vi "Buffer CORE.vi"(5 "Parameters":T3={"Index"=0, "Size"=3000, "Samples"=0, "Ordered ?"=FALSE}, 7 "Mode":T2, 8 "Error IN":errorcluster, 10 "DATA IN":T1[](array[typedef])) -> (0 "Error OUT":errorcluster, 2 "DATA OUT":T1[](array[typedef]), 3 "New Element ?":bool, 4 "Index":i32)   [LabVIEW 2017, in "PMU data buffer.lvlib"]
uses:
  PMU data buffer.lvlib
  Buffer Settings.ctl
  Buffer state.ctl
  Buffer DATA cluster.ctl
panel:
  # "Buffer Paremeters"
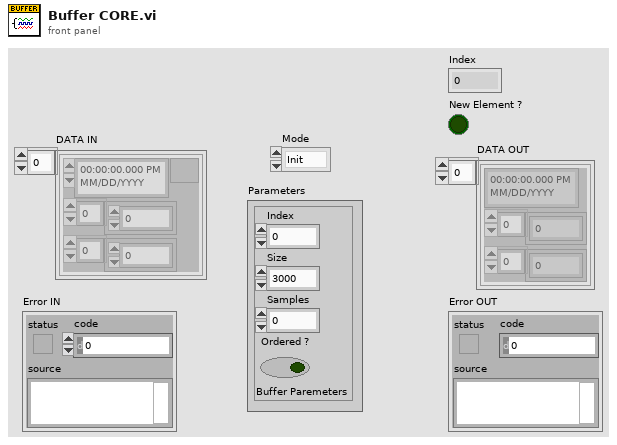
[diagram p1: front panel]
types:
  T1 = typedef "PMU data buffer.lvlib/Buffer DATA cluster.ctl" = cluster{timestamp, csg[], sgl[]}
  T2 = typedef "PMU data buffer.lvlib/Buffer state.ctl" = enum16{"Init", "Change Size", "Flush", "Exit", "Add", "Get", "Hist_Toggle", "Add_Serv"}
  T3 = typedef "PMU data buffer.lvlib/Buffer Settings.ctl" = cluster{"Index":i32, "Size":i32, "Samples":i32, "Ordered ?":bool}
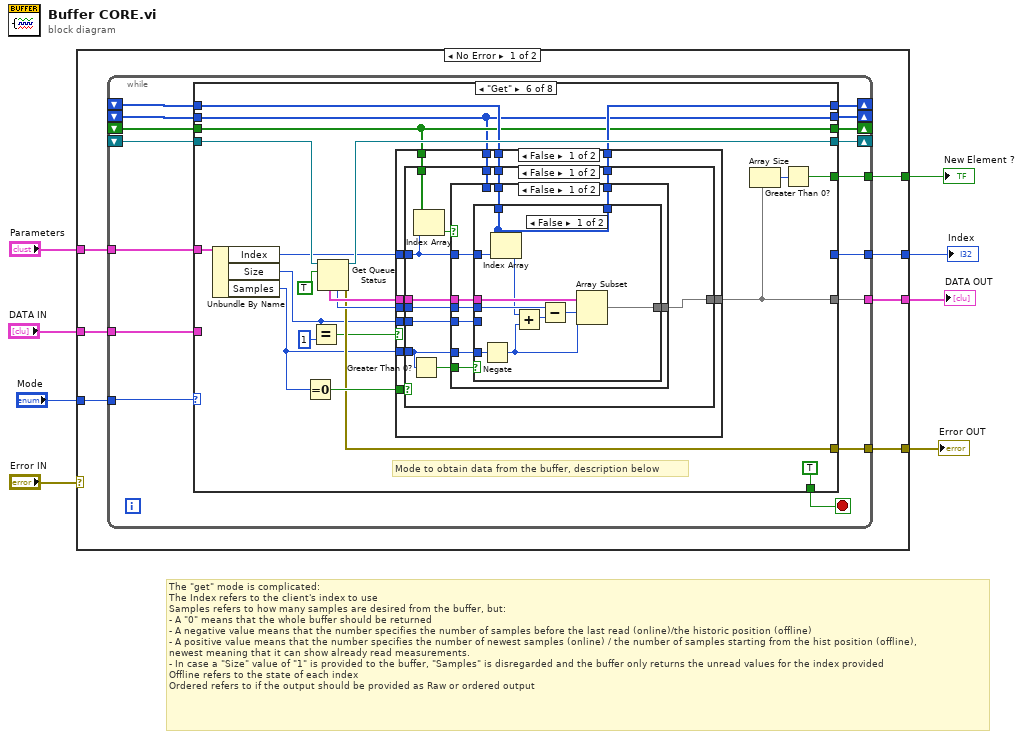
[diagram p0: block diagram]
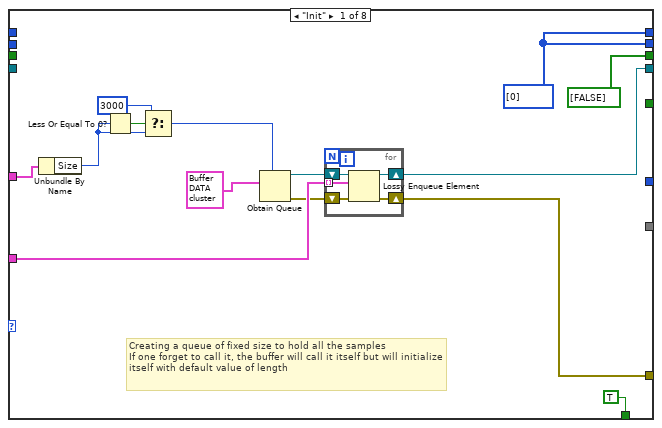
[diagram p2: hidden frame]
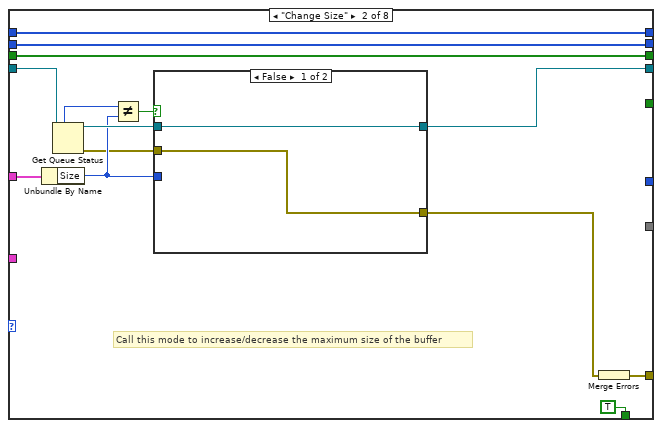
[diagram p3: hidden frame]
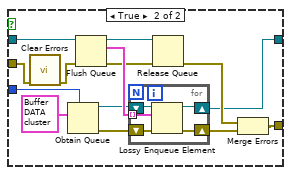
[diagram p4: hidden frame]
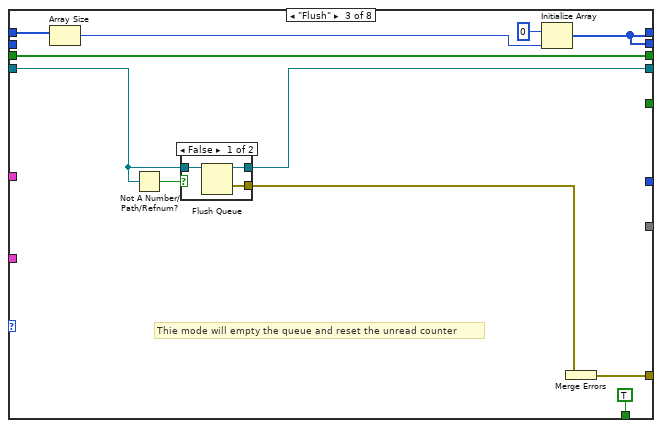
[diagram p5: hidden frame]
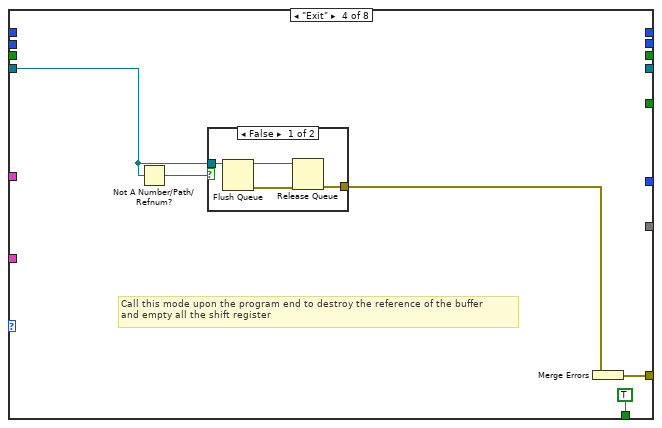
[diagram p7: hidden frame]
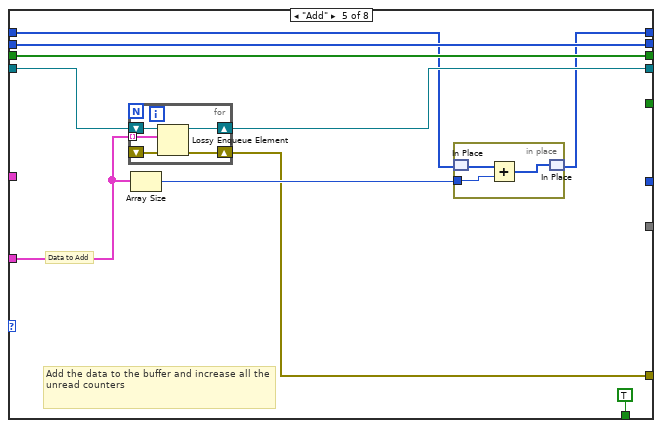
[diagram p9: hidden frame]
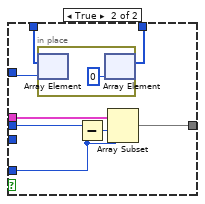
[diagram p10: hidden frame]
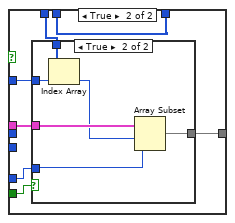
[diagram p11: hidden frame]
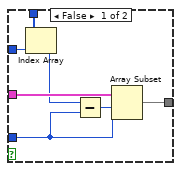
[diagram p12: hidden frame]
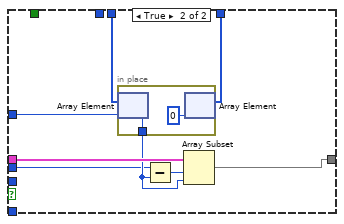
[diagram p14: hidden frame]
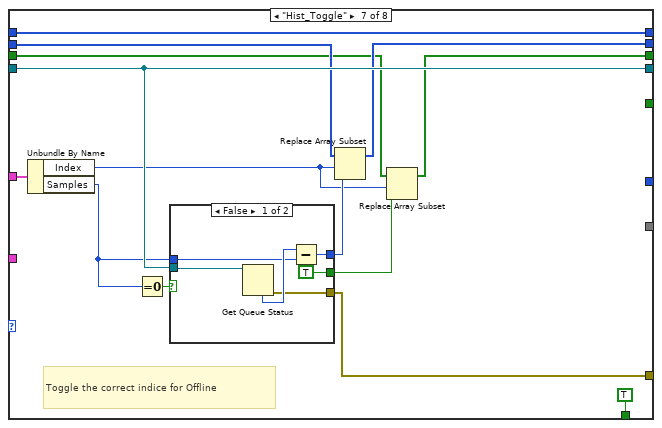
[diagram p15: hidden frame]
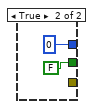
[diagram p16: hidden frame]
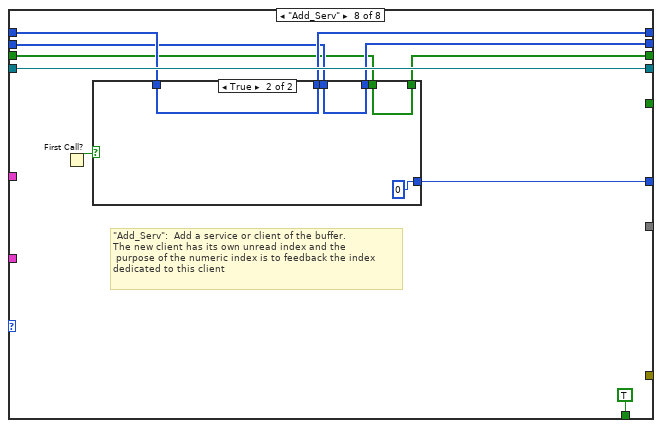
[diagram p17: hidden frame]
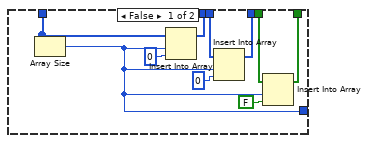
[diagram p18: hidden frame]
diagram:
  # "The \"get\" mode is complicated:\nThe Index refers to the client's index to use\nSamples refers to how many samples are desired from the buffer, but:\n- A \"0\" means that the whole buffer should be returned\n- A negative value means that the number specifies the number of samples before the last read (online)/the historic position (offline)\n- A positive value means that the number specifies the number of newest samples (online) / the number of samples starting from the hist position (offline), \nnewest meaning that it can show already read measurements. \n- In case a \"Size\" value of \"1\" is provided to the buffer, \"Samples\" is disregarded and the buffer only returns the unread values for the index provided\nOffline refers to the state of each index\nOrdered refers to if the output should be provided as Raw or ordered output"
  n1 = case shown="No Error" "Error IN" {
    selector: "Error IN" -> [_ w278]
    tunnel: "Mode" -> [w15 _]
    tunnel: [w10 w278] -> w8
    tunnel: "DATA IN" -> [w14 _]
    tunnel: "Parameters" -> [w13 _]
    tunnel: [w12 _] -> w4
    tunnel: [w11 _] -> w1
    tunnel: [w9 _] -> w3
    frame No Error {
      n2 = while {
        tunnel: w15 -> [w16]
        tunnel: w14 -> [w31]
        tunnel: w13 -> [w29]
        shift-right: [w27] -> _
        shift-left: _ -> [w28]
        tunnel: [w26] -> w12
        tunnel: [w25] -> w11
        shift-right: [w24] -> _
        shift-left: _ -> [w23]
        tunnel: [w22] -> w10
        shift-right: [w20] -> _
        shift-left: _ -> [w21]
        shift-right: [w18] -> _
        shift-left: _ -> [w19]
        tunnel: [w17] -> w9
        stop <- w30 stop-if-true
        n3 = case shown="\"Get\"" w16 {
          tunnel: w31 -> [w43 _ _ _ w118 _ _ _]
          tunnel: [TRUE TRUE TRUE TRUE TRUE TRUE TRUE TRUE] -> w30
          tunnel: w29 -> [w42 w63 _ _ _ w142 w241 _]
          tunnel: w28 -> [_ w60 w89 _ w111 w141 w244 w261]
          tunnel: [w40 w60 w88 _ w110 w138 w244 w260] -> w27
          tunnel: [_ _ _ _ _ w136 _ _] -> w26
          tunnel: [_ _ _ _ _ w131 _ _] -> w25
          tunnel: [w41 w57 w95 _ w115 w144 w242 w262] -> w24
          tunnel: w23 -> [_ w56 w92 w101 w117 w146 w242 w262]
          tunnel: [w38 w62 w93 w104 w112 w133 w232 _] -> w22
          tunnel: w21 -> [_ w59 _ _ w113 w134 w239 w259]
          tunnel: [w40 w59 w88 _ w113 w134 w238 w258] -> w20
          tunnel: w19 -> [_ w58 w90 _ w116 w135 w236 w257]
          tunnel: [bool[] [FALSE] w58 w90 _ w116 w135 w235 w256] -> w18
          tunnel: [_ _ _ _ _ _ _ w255] -> w17
          frame "Init" {
            w40 = i32[] [0]
            # "Creating a queue of fixed size to hold all the samples\nIf one forget to call it, the buffer will call it itself but will initialize itself with default value of length"
            n4 = Unbundle By Name(w42) -> ("Size"=w33:i32)
            n5 = Less Or Equal To 0?(x=w33) -> (x <= 0?=w34:bool)
            n6 = Select(t=3000, s=w34, f=w33) -> (s? t:f=w35:i32)
            n7 = Obtain Queue(max queue size (-1, unlimited)=w35, element data type=T1 {timestamp(0 s since 1904-01-01), [], []}) -> (queue out=w44:refnum<queue>, error out=w39:errorcluster)  [unwired: 3 in, 1 out]
            n8 = for {
              tunnel: w43 -> [w49] mode=indexing
              shift-right: [w48] -> w41
              shift-left: w44 -> [w50]
              shift-right: [w47] -> w38
              shift-left: w39 -> [w46]
              n9 = Lossy Enqueue Element(queue=w50, element=w49, error in (no error)=w46) -> (queue out=w48:refnum<queue>, error out=w47:errorcluster)  [unwired: 2 out]
            }
          }
          frame "Change Size" {
            # "Call this mode to increase/decrease the maximum size of the buffer"
            n10 = Unbundle By Name(w63) -> ("Size"=w53:i32)
            n11 = Get Queue Status(queue=w56) -> (queue out=w55:refnum<queue>, max queue size=w54:i32, error out=w51:errorcluster)  [unwired: 2 in, 5 out]
            n12 = Not Equal?(x=w54, y=w53) -> (x != y?=w52:bool)
            n13 = case shown="False" w52 {
              tunnel: [w65 w69] -> w61
              tunnel: [w66 w77] -> w57
              tunnel: w55 -> [w66 w74]
              tunnel: w53 -> [_ w73]
              tunnel: w51 -> [w65 w68]
              frame False {
              }
              frame True {
                n14 = call <vilib>:"Clear Errors.vi"("error in (no error)"=w68) -> ("error out"=w67:errorcluster)  [unwired: 5 in, 1 out]
                n15 = Obtain Queue(max queue size (-1, unlimited)=w73, element data type=T1 {timestamp(0 s since 1904-01-01), [], []}) -> (queue out=w76:refnum<queue>, error out=w79:errorcluster)  [unwired: 3 in, 1 out]
                n16 = Flush Queue(queue=w74, error in (no error)=w67) -> (queue out=w72:refnum<queue>, remaining elements=w80:T1[], error out=w71:errorcluster)
                n17 = for {
                  tunnel: w80 -> [w83] mode=indexing
                  shift-right: [w84] -> w77
                  shift-left: w76 -> [w85]
                  shift-right: [w81] -> w70
                  shift-left: w79 -> [w82]
                  n18 = Lossy Enqueue Element(queue=w85, element=w83, error in (no error)=w82) -> (queue out=w84:refnum<queue>, error out=w81:errorcluster)  [unwired: 2 out]
                }
                n19 = Release Queue(queue=w72, error in (no error)=w71) -> (error out=w78:errorcluster)  [unwired: 1 in, 2 out]
                n20 = Merge Errors(w78, w70) -> (w69:errorcluster)
              }
            }
            n21 = Merge Errors(w61) -> (w62:errorcluster)
          }
          frame "Flush" {
            # "Thie mode will empty the queue and reset the unread counter"
            n22 = Array Size(array=w89) -> (size(s)=w87:i32)
            n23 = Not A Number/Path/Refnum?(number/path/refnum=w92) -> (NaN/Path/Refnum?=w91:bool)
            n24 = case shown="False" w91 {
              tunnel: w92 -> [w99 w100]
              tunnel: [w98 w100] -> w95
              tunnel: [w97 _] -> w94
              frame False {
                n25 = Flush Queue(queue=w99) -> (queue out=w98:refnum<queue>, error out=w97:errorcluster)  [unwired: 1 in, 1 out]
              }
              frame True {
              }
            }
            n26 = Initialize Array(0 ("size(s)"), w87) -> (w88:i32[])
            n27 = Merge Errors(w94) -> (w93:errorcluster)
          }
          frame "Exit" {
            # "Call this mode upon the program end to destroy the reference of the buffer\nand empty all the shift register"
            n28 = Not A Number/Path/Refnum?(number/path/refnum=w101) -> (NaN/Path/Refnum?=w102:bool)
            n29 = case shown="False" w102 {
              tunnel: w101 -> [w109 _]
              tunnel: [w106 _] -> w103
              frame False {
                n30 = Flush Queue(queue=w109) -> (queue out=w107:refnum<queue>, error out=w108:errorcluster)  [unwired: 1 in, 1 out]
                n31 = Release Queue(queue=w107, error in (no error)=w108) -> (error out=w106:errorcluster)  [unwired: 1 in, 2 out]
              }
              frame True {
              }
            }
            n32 = Merge Errors(w103) -> (w104:errorcluster)
          }
          frame "Add" {
            # "Add the data to the buffer and increase all the unread counters"
            # "Data to Add"
            n33 = for {
              tunnel: w118 -> [w125] mode=indexing
              shift-right: [w123] -> w112
              shift-left: _ -> [w124]
              shift-right: [w126] -> w115
              shift-left: w117 -> [w127]
              n34 = Lossy Enqueue Element(queue=w127, element=w125, error in (no error)=w124) -> (queue out=w126:refnum<queue>, error out=w123:errorcluster)  [unwired: 2 out]
            }
            n35 = Array Size(array=w118) -> (size(s)=w114:i32)
            n36 = in-place {
              in-place-border: w114 -> [w122]
              n37 = in-place-match #1(w111) -> (w120:i32[])
              n38 = Add(x=w120, y=w122) -> (x+y=w121:i32[])
              n39 = in-place-match #1(w121) -> (w110:i32[])
            }
          }
          frame "Get" {
            # "Mode to obtain data from the buffer, description below"
            n40 = Unbundle By Name(w142) -> ("Index"=w140:i32, "Size"=w129:i32, "Samples"=w132:i32)
            n41 = Equal To 0?(x=w132) -> (x = 0?=w139:bool)
            n42 = Equal?(x=w129, y=1) -> (x = y?=w128:bool)
            n43 = Get Queue Status(queue=w146, return elements? (F)=TRUE) -> (queue out=w144:refnum<queue>, error out=w133:errorcluster, # elements in queue=w143:i32, elements=w145:T1[])  [unwired: 1 in, 4 out]
            n44 = case shown="False" w128 {
              tunnel: w145 -> [w159 w227]
              tunnel: w143 -> [w158 w222]
              tunnel: w141 -> [w157 w229]
              tunnel: w140 -> [w156 w223]
              tunnel: w139 -> [w155 _]
              tunnel: [w154 w228] -> w138
              tunnel: w135 -> [w153 _]
              tunnel: w134 -> [w152 _]
              tunnel: w132 -> [w151 _]
              tunnel: [w150 w226] -> w131
              tunnel: w129 -> [w149 _]
              frame False {
                n45 = case shown="False" w155 {
                  tunnel: w159 -> [w171 w221]
                  tunnel: [w170 w221] -> w150
                  tunnel: w158 -> [w169 _]
                  tunnel: w157 -> [w168 w220]
                  tunnel: w156 -> [w162 _]
                  tunnel: w151 -> [w166 _]
                  tunnel: [w165 w220] -> w154
                  tunnel: w153 -> [w163 _]
                  tunnel: w152 -> [w161 _]
                  tunnel: w149 -> [w160 _]
                  frame False {
                    n46 = Greater Than 0?(x=w166) -> (x > 0?=w167:bool)
                    n47 = Index Array(array=w163, index=w162) -> (element=w164:bool)
                    n48 = case shown="False" w164 {
                      tunnel: w171 -> [w180 w203]
                      tunnel: [w179 w200] -> w170
                      tunnel: w169 -> [w178 _]
                      tunnel: w168 -> [w177 w201]
                      tunnel: w162 -> [w176 w206]
                      tunnel: w167 -> [w175 w205]
                      tunnel: w166 -> [w174 w204]
                      tunnel: [w173 w201] -> w165
                      tunnel: w161 -> [_ w202]
                      tunnel: w160 -> [w172 _]
                      frame False {
                        n49 = case shown="False" w175 {
                          tunnel: w180 -> [w190 w196]
                          tunnel: [w189 w195] -> w179
                          tunnel: w178 -> [w187 w197]
                          tunnel: w177 -> [w182 w193]
                          tunnel: w176 -> [w184 w194]
                          tunnel: w174 -> [w183 w191]
                          tunnel: [w182 w192] -> w173
                          tunnel: w172 -> [_ _]
                          frame False {
                            n50 = Negate(x=w183) -> (-x=w181:i32)
                            n51 = Index Array(array=w182, index=w184) -> (element=w185:i32)
                            n52 = Add(x=w185, y=w181) -> (x+y=w186:i32)
                            n53 = Subtract(x=w187, y=w186) -> (x-y=w188:i32)
                            n54 = Array Subset(array=w190, index=w188, length=w181) -> (w189:T1[])
                          }
                          frame True {
                            n55 = in-place {
                              n56 = in-place-array #2(w193, w194) -> ()  [unwired: 1 out]
                              n57 = in-place-array #2(0 ("new element/subarray")) -> (w192:i32[])  [unwired: 1 out]
                            }
                            n58 = Subtract(x=w197, y=w191) -> (x-y=w198:i32)
                            n59 = Array Subset(array=w196, index=w198, length=w191) -> (w195:T1[])
                          }
                        }
                      }
                      frame True {
                        n60 = case shown="True" w205 {
                          tunnel: w203 -> [w213 w219]
                          tunnel: [w212 w217] -> w200
                          tunnel: w202 -> [w209 w216]
                          tunnel: w206 -> [w210 w215]
                          tunnel: w204 -> [w207 w218]
                          frame False {
                            n61 = Index Array(array=w209, index=w210) -> (element=w208:i32)
                            n62 = Subtract(x=w208, y=w207) -> (x-y=w211:i32)
                            n63 = Array Subset(array=w213, index=w211, length=w207) -> (w212:T1[])
                          }
                          frame True {
                            n64 = Index Array(array=w216, index=w215) -> (element=w214:i32)
                            n65 = Array Subset(array=w219, index=w214, length=w218) -> (w217:T1[])
                          }
                        }
                      }
                    }
                  }
                  frame True {
                  }
                }
              }
              frame True {
                n66 = in-place {
                  in-place-border: [w230] -> w224
                  n67 = in-place-array #3(w229, w223) -> (w230:i32)
                  n68 = in-place-array #3(0 ("new element/subarray")) -> (w228:i32[])  [unwired: 1 out]
                }
                n69 = Subtract(x=w222, y=w224) -> (x-y=w225:i32)
                n70 = Array Subset(array=w227, index=w225, length=w224) -> (w226:T1[])
              }
            }
            n71 = Array Size(array=w131) -> (size(s)=w137:i32)
            n72 = Greater Than 0?(x=w137) -> (x > 0?=w136:bool)
          }
          frame "Hist_Toggle" {
            # "Toggle the correct indice for Offline"
            n73 = Unbundle By Name(w241) -> ("Index"=w233:i32, "Samples"=w240:i32)
            n74 = Equal To 0?(x=w240) -> (x = 0?=w243:bool)
            n75 = case shown="False" w243 {
              tunnel: [TRUE FALSE] -> w234
              tunnel: w240 -> [w248 _]
              tunnel: [w247 0 ("Index")] -> w237
              tunnel: w242 -> [w250 _]
              tunnel: [w246 _] -> w232
              frame False {
                n76 = Get Queue Status(queue=w250) -> (error out=w246:errorcluster, # elements in queue=w249:i32)  [unwired: 2 in, 6 out]
                n77 = Subtract(x=w249, y=w248) -> (x-y=w247:i32)
              }
              frame True {
              }
            }
            n78 = Replace Array Subset(array=w239, new element=w237, index=w233) -> (w238:i32[])
            n79 = Replace Array Subset(array=w236, new element=w234, index=w233) -> (w235:bool[])
          }
          frame "Add_Serv" {
            # "\"Add_Serv\":  Add a service or client of the buffer. \nThe new client has its own unread index and the\n purpose of the numeric index is to feedback the index \ndedicated to this client"
            n80 = First Call?() -> (First Call?: T/F=w254:bool)
            n81 = case shown="True" w254 {
              tunnel: w261 -> [w264 w277]
              tunnel: [w273 w277] -> w260
              tunnel: w259 -> [w272 w276]
              tunnel: [w271 w276] -> w258
              tunnel: w257 -> [w270 w275]
              tunnel: [w269 w275] -> w256
              tunnel: [w265 0] -> w255
              frame False {
                n82 = Array Size(array=w264) -> (size(s)=w265:i32)
                n83 = Insert Into Array(array=w264, index=w265, new element=0 ("new element/subarray")) -> (w273:i32[])
                n84 = Insert Into Array(array=w272, index=w265, new element=0 ("new element/subarray")) -> (w271:i32[])
                n85 = Insert Into Array(array=w270, index=w265, new element=FALSE ("new element/subarray")) -> (w269:bool[])
              }
              frame True {
              }
            }
          }
        }
      }
    }
    frame Error {
    }
  }
  "Error OUT" <- w8
  "New Element ?" <- w4
  "Index" <- w3
  "DATA OUT" <- w1
